vi "Anritsu VNA Set Start and Stop Frequencies.vi"(6 "Channel":i8=1 min=1 step=1, 7 "Anritsu VNA":T1, 8 "error in (no error)":errorcluster, 10 "Start/Stop Freqs, MHz":cluster{"Fstart":dbl, "Fstop":dbl}, 11 "VISA Resource Name":refnum<visa-resource-name>) -> (0 "error out":errorcluster, 3 "dup VISA Resource Name":refnum<visa-resource-name>)   [LabVIEW 2011]
doc: "This VI for the HP 8753B is used to read the number of stimulus points."
uses:
  TypeDefs/Anritsu VNA Instrument Info.ctl
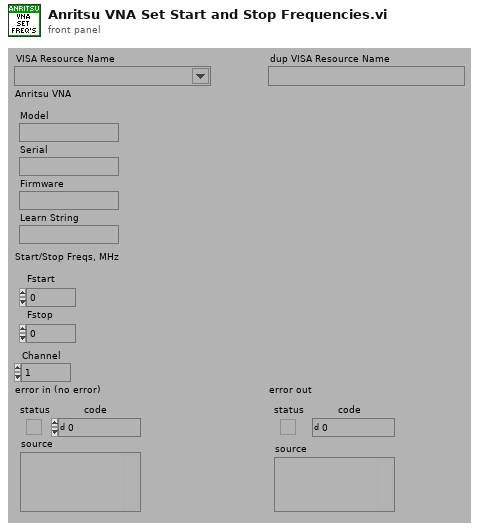
[diagram p1: front panel]
types:
  T1 = typedef "Anritsu VNA Instrument Info.ctl" = cluster{"Model":string, "Serial":string, "Firmware":string, "Learn String":string}
  T2 = typedef "Anritsu VNA Model.ctl" = enum16{"Not Supported", "37XXXX", "MS20XXX", "MS462XX", "MS464XX"}
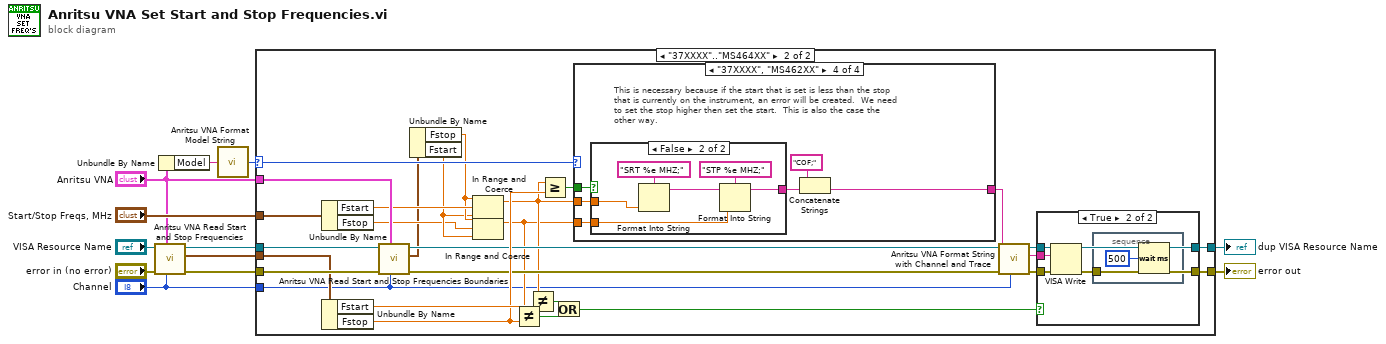
[diagram p0: block diagram]
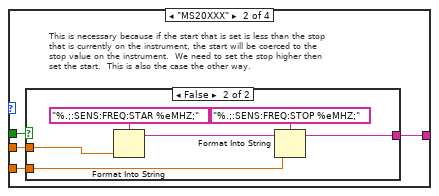
[diagram p4: hidden frame]
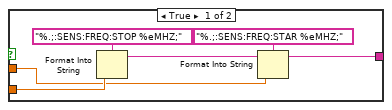
[diagram p5: hidden frame]
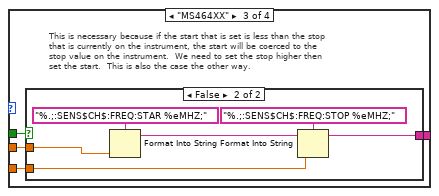
[diagram p6: hidden frame]
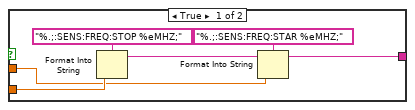
[diagram p7: hidden frame]
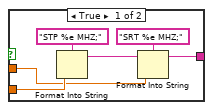
[diagram p8: hidden frame]
diagram:
  n1 = call "Anritsu VNA Read Start and Stop Frequencies.vi"("Channel"="Channel", "Anritsu VNA"="Anritsu VNA", "error in (no error)"="error in (no error)", "VISA Resource Name"="VISA Resource Name") -> ("error out"=w7:errorcluster, "Start/Stop Freqs, MHz"=w5:cluster{"Fstart":dbl, "Fstop":dbl}, "dup VISA Resource Name"=w6:refnum<visa-resource-name>)  [unwired: 5 out]
  n2 = Unbundle By Name("Anritsu VNA") -> ("Model"=w4:string)
  n3 = call "Anritsu VNA Format Model String.vi"("Model"=w4) -> ("Model"=w3:T2)
  n4 = case shown="\"37XXXX\"..\"MS464XX\"" w3 {
    selector: w3 -> [_ w31]
    tunnel: [w14 w40] -> w12
    tunnel: [w13 w39] -> w11
    tunnel: "Start/Stop Freqs, MHz" -> [_ w38]
    tunnel: w7 -> [w13 w29]
    tunnel: w6 -> [w14 w30]
    tunnel: w5 -> [_ w19]
    tunnel: "Anritsu VNA" -> [_ w26]
    tunnel: "Channel" -> [_ w15]
    frame "Not Supported" {
    }
    frame "37XXXX".."MS464XX" {
      n5 = Unbundle By Name(w38) -> ("Fstart"=w25:dbl, "Fstop"=w21:dbl)
      n6 = Unbundle By Name(w19) -> ("Fstart"=w37:dbl, "Fstop"=w32:dbl)
      n7 = call "Anritsu VNA Read Start and Stop Frequencies Boundaries.vi"("Channel"=w15, "Anritsu VNA"=w26, "error in (no error)"=w29, "VISA Resource Name"=w30) -> ("error out"=w28:errorcluster, "Start/Stop Freq Bounds, MHz"=w18:cluster{"Fstart":dbl, "Fstop":dbl}, "dup VISA Resource Name"=w27:refnum<visa-resource-name>)  [unwired: 5 out]
      n8 = Unbundle By Name(w18) -> ("Fstop"=w23:dbl, "Fstart"=w22:dbl)
      n9 = In Range and Coerce(upper limit=w23, x=w25, lower limit=w22) -> (coerced(x)=w24:dbl)  [unwired: 1 out]
      n10 = In Range and Coerce(upper limit=w23, x=w21, lower limit=w22) -> (coerced(x)=w20:dbl)  [unwired: 1 out]
      n11 = Not Equal?(x=w20, y=w32) -> (x != y?=w35:bool)
      n12 = Not Equal?(x=w24, y=w37) -> (x != y?=w36:bool)
      n13 = Greater Or Equal?(x=w24, y=w32) -> (x >= y?=w33:bool)
      n14 = Or(x=w36, y=w35) -> (x .or. y?=w34:bool)
      n15 = case shown="\"37XXXX\", \"MS462XX\"" w31 {
        tunnel: [_ w44 w60 w75] -> w17
        tunnel: w24 -> [_ w43 w59 w78]
        tunnel: w20 -> [_ w42 w58 w77]
        tunnel: w33 -> [_ w41 w57 w76]
        frame "Not Supported" {
        }
        frame "MS20XXX" {
          # "This is necessary because if the start that is set is less than the stop\nthat is currently on the instrument, the start will be coerced to the\nstop value on the instrument.  We need to set the stop higher then\nset the start.  This is also the case the other way."
          n16 = case shown="False" w41 {
            tunnel: [w50 w56] -> w44
            tunnel: w43 -> [w45 w55]
            tunnel: w42 -> [w46 w54]
            frame True {
              n17 = Format Into String(format string="%.;:SENS:FREQ:STOP %eMHZ;", w46) -> (resulting string=w47:string)  [unwired: 2 in, 1 out]
              n18 = Format Into String(format string="%.;:SENS:FREQ:STAR %eMHZ;", initial string=w47, w45) -> (resulting string=w50:string)  [unwired: 1 in, 1 out]
            }
            frame False {
              n19 = Format Into String(format string="%.;:SENS:FREQ:STAR %eMHZ;", w55) -> (resulting string=w51:string)  [unwired: 2 in, 1 out]
              n20 = Format Into String(format string="%.;:SENS:FREQ:STOP %eMHZ;", initial string=w51, w54) -> (resulting string=w56:string)  [unwired: 1 in, 1 out]
            }
          }
        }
        frame "MS464XX" {
          # "This is necessary because if the start that is set is less than the stop\nthat is currently on the instrument, the start will be coerced to the\nstop value on the instrument.  We need to set the stop higher then\nset the start.  This is also the case the other way."
          n21 = case shown="False" w57 {
            tunnel: [w66 w72] -> w60
            tunnel: w59 -> [w61 w71]
            tunnel: w58 -> [w62 w70]
            frame True {
              n22 = Format Into String(format string="%.;:SENS:FREQ:STOP %eMHZ;", w62) -> (resulting string=w63:string)  [unwired: 2 in, 1 out]
              n23 = Format Into String(format string="%.;:SENS:FREQ:STAR %eMHZ;", initial string=w63, w61) -> (resulting string=w66:string)  [unwired: 1 in, 1 out]
            }
            frame False {
              n24 = Format Into String(format string="%.;:SENS$CH$:FREQ:STAR %eMHZ;", w71) -> (resulting string=w67:string)  [unwired: 2 in, 1 out]
              n25 = Format Into String(format string="%.;:SENS$CH$:FREQ:STOP %eMHZ;", initial string=w67, w70) -> (resulting string=w72:string)  [unwired: 1 in, 1 out]
            }
          }
        }
        frame "37XXXX", "MS462XX" {
          # "This is necessary because if the start that is set is less than the stop\nthat is currently on the instrument, an error will be created.  We need\nto set the stop higher then set the start.  This is also the case the\nother way."
          n26 = case shown="False" w76 {
            tunnel: [w84 w90] -> w74
            tunnel: w78 -> [w79 w89]
            tunnel: w77 -> [w80 w88]
            frame True {
              n27 = Format Into String(format string="STP %e MHZ;", w80) -> (resulting string=w81:string)  [unwired: 2 in, 1 out]
              n28 = Format Into String(format string="SRT %e MHZ;", initial string=w81, w79) -> (resulting string=w84:string)  [unwired: 1 in, 1 out]
            }
            frame False {
              n29 = Format Into String(format string="SRT %e MHZ;", w89) -> (resulting string=w85:string)  [unwired: 2 in, 1 out]
              n30 = Format Into String(format string="STP %e MHZ;", initial string=w85, w88) -> (resulting string=w90:string)  [unwired: 1 in, 1 out]
            }
          }
          n31 = Concatenate Strings("COF;", w74) -> (w75:string)
        }
      }
      n32 = call "Anritsu VNA Format String with Channel and Trace.vi"("Channel"=w15, "String"=w17) -> ("String Out"=w16:string)  [unwired: 1 in, 6 out]
      n33 = case shown="True" w34 {
        tunnel: [w92 w97] -> w40
        tunnel: [w91 w93] -> w39
        tunnel: w16 -> [_ w96]
        tunnel: w28 -> [w91 w95]
        tunnel: w27 -> [w92 w94]
        frame False {
        }
        frame True {
          n34 = VISA Write(VISA resource name=w94, write buffer=w96, error in (no error)=w95) -> (VISA resource name out=w97:refnum<visa-resource-name>, error out=w93:errorcluster)  [unwired: 1 out]
          n35 = stacked-sequence {
            tunnel: w93 -> [_]
            frame #0 {
              n36 = Wait (ms)(milliseconds to wait=u32 500) -> ()  [unwired: 1 out]
            }
          }
        }
      }
    }
  }
  "dup VISA Resource Name" <- w12
  "error out" <- w11
